vi "Create Prefix.vi"() -> (2 "Text":string)   [LabVIEW 2018, in "IV_data.lvclass"]
uses:
  IV_data.lvclass
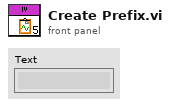
[diagram p1: front panel]
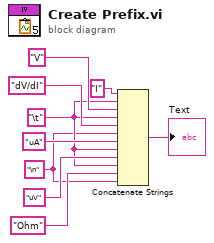
[diagram p0: block diagram]
diagram:
  w2 = "\n"
  w4 = "\t" ("string")
  n1 = Concatenate Strings("I" ("nameX"), w4, "V" ("nameY"), w4, "dV/dI" ("namedYdX"), w2, "uA" ("unitX"), w4, "uV" ("unitY"), w4, "Ohm" ("unitdYdX"), w2) -> (→"Text":string)
